vi "0x06PresetSingleRegister.vi"(6 "Data":u16, 8 "error in (no error)":errorcluster, 9 "Register":u16, 10 "Addressc":u8, 11 "RTU in":refnum<class "RTU.lvclass">) -> (0 "error out":errorcluster, 2 "Frame":string, 3 "RTU out":refnum<class "RTU.lvclass">)   [LabVIEW 2017, in "ModBUS.lvlib" / "RTU.lvclass"]
uses:
  RTU.lvclass
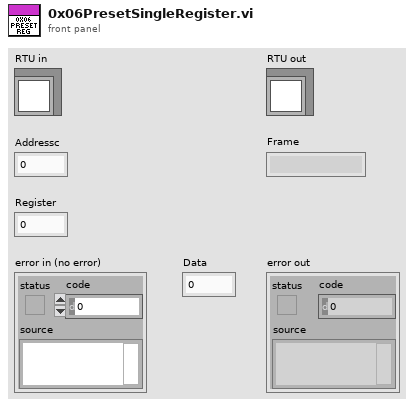
[diagram p1: front panel]
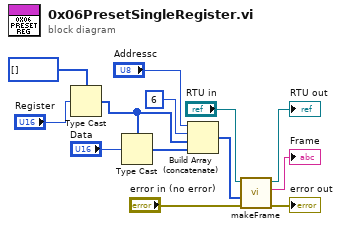
[diagram p0: block diagram]
diagram:
  n1 = Type Cast(type=u8[] [], x="Register") -> (*(type *) &x=w12:u8[])
  n2 = Type Cast(type=w12, x="Data") -> (*(type *) &x=w11:u8[])
  n3 = Build Array (concatenate)("Addressc", u8 6 ("element"), w12, w11) -> (w10:u8[])
  n4 = call-dynamic "makeFrame.vi"("error in (no error)"="error in (no error)", "Data"=w10, "RTU in"="RTU in") -> ("error out"=→"error out":errorcluster, "Frame"=→"Frame":string, "RTU out"=→"RTU out":refnum<class "RTU.lvclass">)  [unwired: 6 in]
